vi "Read (Single Point).vi"(0 "VISA resource name":refnum<visa-resource-name>, 11 "error in (no error)":errorcluster) -> (4 "VISA resource name out":refnum<visa-resource-name>, 6 "Measurement":dbl, 15 "error out":errorcluster)   [LabVIEW 2021, in "Agilent 34420.lvlib"]
doc: "Reads and returns a single measurement from the instrument.\n\n<B>Note:</B>\n\nChanges the <B>Trigger Source</B> to immediate and takes a measurement immediately."
uses:
  <instrlib>/Agilent 34420/Agilent 34420.lvlib
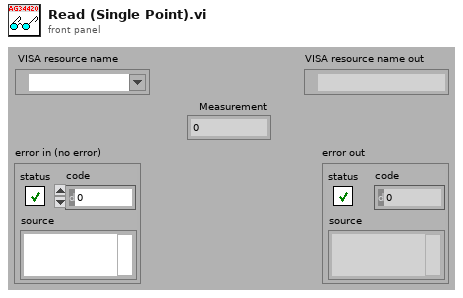
[diagram p1: front panel]
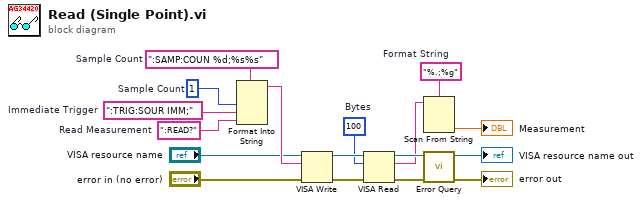
[diagram p0: block diagram]
diagram:
  w1 = 1  # Sample Count
  w5 = ":TRIG:SOUR IMM;"  # Immediate Trigger
  w7 = ":SAMP:COUN %d;%s%s"  # Sample Count
  w6 = ":READ?"  # Read Measurement
  w9 = "%.;%g"  # Format String
  w15 = u32 100  # Bytes
  n1 = Format Into String(format string=w7, w1, w5, w6) -> (resulting string=w4:string)  [unwired: 2 in, 1 out]
  n2 = VISA Write(VISA resource name="VISA resource name", write buffer=w4, error in (no error)="error in (no error)") -> (VISA resource name out=w16:refnum<visa-resource-name>, error out=w17:errorcluster)  [unwired: 1 out]
  n3 = VISA Read(VISA resource name=w16, byte count=w15, error in (no error)=w17) -> (VISA resource name out=w14:refnum<visa-resource-name>, read buffer=w10:string, error out=w13:errorcluster)  [unwired: 1 out]
  n4 = Scan From String(format string=w9, input string=w10) -> (output 1=→"Measurement":dbl)  [unwired: 3 in, 3 out]
  n5 = call <instrlib>:"Error Query.vi"("error in (no error)"=w13, "VISA resource name"=w14) -> ("error out"=→"error out":errorcluster, "VISA resource name out"=→"VISA resource name out":refnum<visa-resource-name>)  [unwired: 6 in, 2 out]
